vi "Atoms to POSCAR.vi"(10 "Volume Factor":dbl=1.0, 11 "Atomic Structure":T1={"Structure Name"="ATK-generated POSCAR  \r\n", "Lattice vector a"=[6.48, 0.0, 0.0], "Lattice vector b"=[0.0, 6.48, 0.0], "Lattice vector c"=[0.0, 0.0, 32.4], "Atoms Array"=[{"Atom Name"="", "Positions (Direct)"=[[0.0, 0.0, 0.0005805493563561], [0.5, 0.5, 0.0005805493563561], [0.5, 0.0, 0.1012044869316679], [0.0, 0.5, 0.1012044869316679], [0.0, 0.0, 0.201657427297086], [0.5, 0.5, 0.201657427297086], [0.5, 0.0, 0.3022756106216986], [0.0, 0.5, 0.3022756106216986], [0.25, 0.25, 0.3937799251008503], [0.75, 0.75, 0.3937799251008503], [0.75, 0.25, 0.5004577122084005], [0.25, 0.75, 0.5004577122084005], [0.0, 0.0, 0.5916454825280393], [0.5, 0.5, 0.5916454825280393], [0.5, 0.0, 0.6986135219684406], [0.0, 0.5, 0.6986135219684406], [0.0, 0.0, 0.7992442554474246], [0.5, 0.5, 0.7992442554474246], [0.5, 0.0, 0.8999316304227629], [0.0, 0.5, 0.8999316304227629]], "Positions (Cartesian)"=[[0.0, 0.0, 0.0005805493563561], [0.5, 0.5, 0.0005805493563561], [0.5, 0.0, 0.1012044869316679], [0.0, 0.5, 0.1012044869316679], [0.0, 0.0, 0.201657427297086], [0.5, 0.5, 0.201657427297086], [0.5, 0.0, 0.3022756106216986], [0.0, 0.5, 0.3022756106216986], [0.25, 0.25, 0.3937799251008503], [0.75, 0.75, 0.3937799251008503], [0.75, 0.25, 0.5004577122084005], [0.25, 0.75, 0.5004577122084005], [0.0, 0.0, 0.5916454825280393], [0.5, 0.5, 0.5916454825280393], [0.5, 0.0, 0.6986135219684406], [0.0, 0.5, 0.6986135219684406], [0.0, 0.0, 0.7992442554474246], [0.5, 0.5, 0.7992442554474246], [0.5, 0.0, 0.8999316304227629], [0.0, 0.5, 0.8999316304227629]]}, {"Atom Name"="", "Positions (Direct)"=[[0.25, 0.25, 0.0508700657751452], [0.75, 0.75, 0.0508700657751452], [0.75, 0.25, 0.1514314226755048], [0.25, 0.75, 0.1514314226755048], [0.25, 0.25, 0.2516943562152962], [0.75, 0.75, 0.2516943562152962], [0.75, 0.25, 0.356312302565805], [0.25, 0.75, 0.356312302565805], [0.0, 0.0, 0.4497768887256497], [0.5, 0.5, 0.4497768887256497], [0.5, 0.0, 0.553935227460559], [0.0, 0.5, 0.553935227460559], [0.25, 0.25, 0.6478094902292927], [0.75, 0.75, 0.6478094902292927], [0.75, 0.25, 0.7489441399571884], [0.25, 0.75, 0.7489441399571884], [0.25, 0.25, 0.8495690683463202], [0.75, 0.75, 0.8495690683463202], [0.75, 0.25, 0.9502664361665122], [0.25, 0.75, 0.9502664361665122]], "Positions (Cartesian)"=[[0.25, 0.25, 0.0508700657751452], [0.75, 0.75, 0.0508700657751452], [0.75, 0.25, 0.1514314226755048], [0.25, 0.75, 0.1514314226755048], [0.25, 0.25, 0.2516943562152962], [0.75, 0.75, 0.2516943562152962], [0.75, 0.25, 0.356312302565805], [0.25, 0.75, 0.356312302565805], [0.0, 0.0, 0.4497768887256497], [0.5, 0.5, 0.4497768887256497], [0.5, 0.0, 0.553935227460559], [0.0, 0.5, 0.553935227460559], [0.25, 0.25, 0.6478094902292927], [0.75, 0.75, 0.6478094902292927], [0.75, 0.25, 0.7489441399571884], [0.25, 0.75, 0.7489441399571884], [0.25, 0.25, 0.8495690683463202], [0.75, 0.75, 0.8495690683463202], [0.75, 0.25, 0.9502664361665122], [0.25, 0.75, 0.9502664361665122]]}], "# of atoms"=40}) -> (3 "POSCAR File":string)   [LabVIEW 2010]
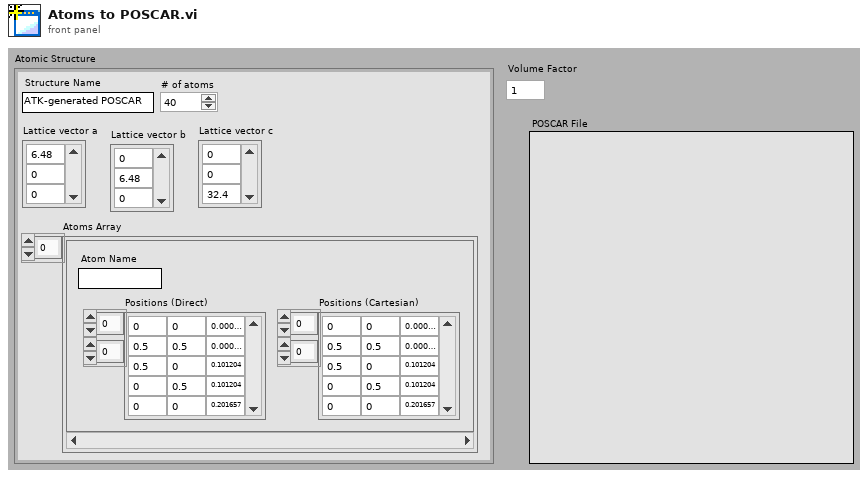
[diagram p1: front panel]
types:
  T1 = cluster{"Structure Name":string, "Lattice vector a":dbl[], "Lattice vector b":dbl[], "Lattice vector c":dbl[], "Atoms Array":cluster{"Atom Name":string, "Positions (Direct)":dbl[][], "Positions (Cartesian)":dbl[][]}[], "# of atoms":i32}
  T2 = cluster{"Atom Name":string, "Positions (Direct)":dbl[][], "Positions (Cartesian)":dbl[][]}[]
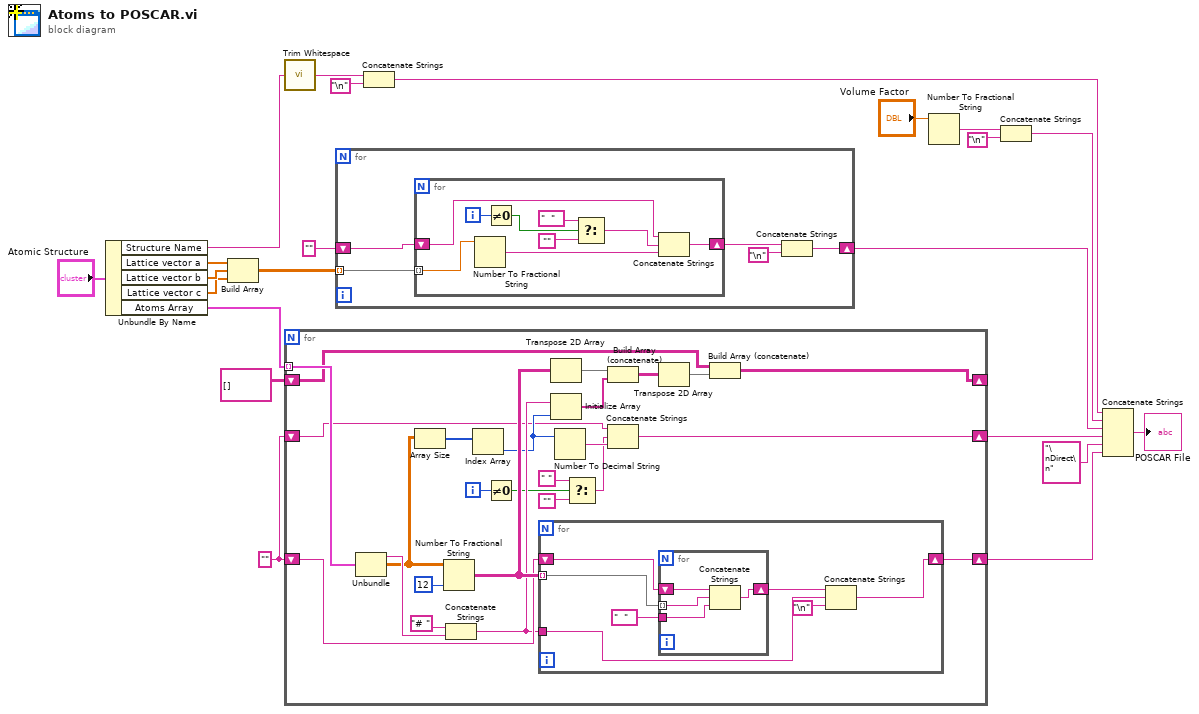
[diagram p0: block diagram]
diagram:
  w9 = ""
  n1 = Unbundle By Name("Atomic Structure") -> ("Structure Name"=w2:string, "Lattice vector a"=w6:dbl[], "Lattice vector b"=w5:dbl[], "Lattice vector c"=w4:dbl[], "Atoms Array"=w3:T2)
  n2 = Build Array(w6, w5, w4) -> (w12:dbl[][])
  n3 = call <vilib>:"Trim Whitespace.vi"("string"=w2) -> ("trimmed string"=w1:string)  [unwired: 1 in]
  n4 = for {
    tunnel: w3 -> [w47] mode=indexing
    shift-right: [w43] -> _
    shift-left: string[][] [] -> [w42]
    shift-right: [w35] -> w20
    shift-left: w9 -> [w34]
    shift-right: [w26] -> w8
    shift-left: w9 -> [w25]
    i -> [w29]
    n5 = Unbundle(w47) -> ("Atom Name"=w46:string, "Positions (Direct)"=w37:dbl[][])  [unwired: 1 out]
    n6 = Array Size(array=w37) -> (size(s)=w44:i32[])
    n7 = Number To Fractional String(number=w37, precision (6)=i16 12) -> (F-format string=w36:string[][])  [unwired: 2 in]
    n8 = Concatenate Strings("# " ("string"), w46) -> (w33:string)
    n9 = Index Array(array=w44) -> (element=w32:i32)  [unwired: 1 in]
    n10 = Not Equal To 0?(x=w29) -> (x != 0?=w31:bool)
    n11 = for {
      tunnel: w36 -> [w54] mode=indexing
      shift-right: [w52] -> w35
      shift-left: w34 -> [w50]
      tunnel: w33 -> [w48]
      n12 = for {
        tunnel: w54 -> [w57] mode=indexing
        shift-right: [w56] -> w49
        shift-left: w50 -> [w55]
        tunnel: "  " ("delimiter (Tab)") -> [w58]
        n13 = Concatenate Strings(w55, w57, w58) -> (w56:string)
      }
      n14 = Concatenate Strings(w49, w48, "\n") -> (w52:string)
    }
    n15 = Transpose 2D Array(2D array=w36) -> (transposed array=w41:string[][])
    n16 = Initialize Array(w33, w32) -> (w40:string[])
    n17 = Number To Decimal String(number=w32) -> (decimal integer string=w28:string)  [unwired: 1 in]
    n18 = Select(t=" " ("string"), s=w31, f="") -> (s? t:f=w27:string)
    n19 = Build Array (concatenate)(w41, w40) -> (w39:string[][])
    n20 = Concatenate Strings(w25, w27, w28) -> (w26:string)
    n21 = Transpose 2D Array(2D array=w39) -> (transposed array=w38:string[][])
    n22 = Build Array (concatenate)(w42, w38) -> (w43:string[][])
  }
  n23 = for {
    shift-right: [w60] -> w10
    shift-left: "" -> [w62]
    tunnel: w12 -> [w63] mode=indexing
    n24 = for {
      shift-right: [w69] -> w61
      shift-left: w62 -> [w70]
      tunnel: w63 -> [w72] mode=indexing
      i -> [w66]
      n25 = Number To Fractional String(number=w72) -> (F-format string=w71:string)  [unwired: 3 in]
      n26 = Not Equal To 0?(x=w66) -> (x != 0?=w65:bool)
      n27 = Select(t="  " ("string"), s=w65, f="") -> (s? t:f=w64:string)
      n28 = Concatenate Strings(w70, w64, w71) -> (w69:string)
    }
    n29 = Concatenate Strings(w61, "\n") -> (w60:string)
  }
  n30 = Concatenate Strings(w1, "\n") -> (w14:string)
  n31 = Number To Fractional String(number="Volume Factor") -> (F-format string=w15:string)  [unwired: 3 in]
  n32 = Concatenate Strings(w15, "\n") -> (w13:string)
  n33 = Concatenate Strings(w14, w13, w10, w8, "\nDirect\n", w20) -> (→"POSCAR File":string)
